vi "Configure Notch Search.vi"(5 "State (T: Enable)":bool=TRUE, 7 "Notch Definition Value (-3.0)":dbl=-3.0, 8 "error in (no error)":errorcluster, 9 "Marker (1)":i32=1, 10 "Channel (1)":i32=1, 11 "VISA resource name":refnum<visa-resource-name>) -> (0 "error out":errorcluster, 3 "VISA resource name out":refnum<visa-resource-name>)   [LabVIEW 2012, in "Tektronix TTR500 Series.lvlib"]
doc: "This VI configure notch marker search."
uses:
  <instrlib>/Tektronix TTR500 Series/Tektronix TTR500 Series.lvlib
panel:
  # "Enable\n\nDisable"
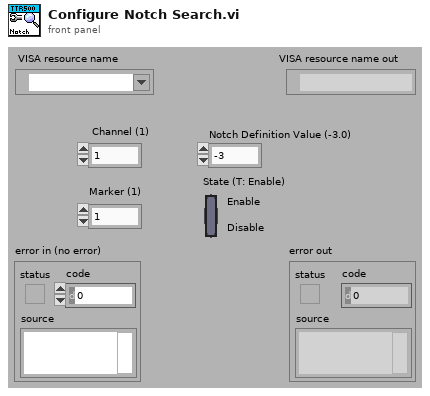
[diagram p1: front panel]
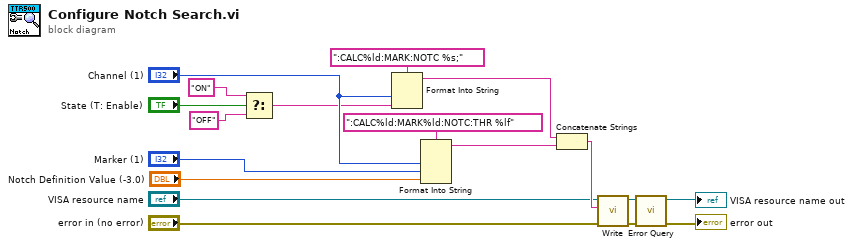
[diagram p0: block diagram]
diagram:
  n1 = Select(t="ON", s="State (T: Enable)", f="OFF") -> (s? t:f=w14:string)
  n2 = Format Into String(format string=":CALC%ld:MARK:NOTC %s;", "Channel (1)", w14) -> (resulting string=w6:string)  [unwired: 2 in, 1 out]
  n3 = Format Into String(format string=":CALC%ld:MARK%ld:NOTC:THR %lf", "Channel (1)", "Marker (1)", "Notch Definition Value (-3.0)") -> (resulting string=w7:string)  [unwired: 2 in, 1 out]
  n4 = Concatenate Strings(w6, w7) -> (w5:string)
  n5 = call <instrlib>:"Write.vi"("error in (no error)"="error in (no error)", "String ()"=w5, "VISA resource name"="VISA resource name") -> ("error out"=w3:errorcluster, "VISA resource name out"=w4:refnum<visa-resource-name>)  [unwired: 6 in, 1 out]
  n6 = call <instrlib>:"Error Query.vi"("error in (no error)"=w3, "VISA resource name"=w4) -> ("error out"=→"error out":errorcluster, "VISA resource name out"=→"VISA resource name out":refnum<visa-resource-name>)  [unwired: 6 in, 2 out]
